vi "PathPlanner_Path_LoadPath.vi"(8 "Reversed":bool, 9 "MaxAcceleration":dbl, 10 "MaxVelocity":dbl, 11 "FileName":string="path1.path") -> (0 "error out":errorcluster, 2 "PathPlannerWayPoints":T10[](array[typedef]) {"HolonomicRotation"."SIN" format="%13.4f"; "HolonomicRotation"."COS" format="%13.4f"; "HolonomicRotation"."VALUE" format="%13.4f"; "NextControl"."Y" format="%14.3f"; "NextControl"."X" format="%14.3f"; "PrevControl"."Y" format="%14.3f"; "PrevControl"."X" format="%14.3f"; "AnchorPoint"."Y" format="%14.3f"; "AnchorPoint"."X" format="%14.3f"}, 3 "PathPlannerPath":T1={"BezierPoints"=[], "PreviewStartingRotation"={"VALUE"=0.0, "COS"=1.0, "SIN"=0.0}, "Reversed"=FALSE, "RotationTargets"=[], "ConstraintZones"=[], "EventMarkers"=[], "GlobalConstraints"={"MaxVelocityMps;"=0.0, "MaxAccelerationMpsSq;"=0.0, "MaxAngularVelRadPsEc;"=0.0, "MaxAngularAccRadPSecSq"=0.0, "Exists"=FALSE}, "GoalEndState"={"Velocity"=0.0, "Rotation"={"VALUE"=0.0, "COS"=1.0, "SIN"=0.0}}, "AllPoints"=[]} {"AllPoints"."HolonomicRotation"."SIN" format="%13.4f"; "AllPoints"."HolonomicRotation"."COS" format="%13.4f"; "AllPoints"."HolonomicRotation"."VALUE" format="%13.4f"; "AllPoints"."Position"."Y" format="%14.3f"; "AllPoints"."Position"."X" format="%14.3f"; "GoalEndState"."Rotation"."SIN" format="%13.4f"; "GoalEndState"."Rotation"."COS" format="%13.4f"; "GoalEndState"."Rotation"."VALUE" format="%13.4f"; "RotationTargets"."target"."SIN" format="%13.4f"; "RotationTargets"."target"."COS" format="%13.4f"; "RotationTargets"."target"."VALUE" format="%13.4f"; "PreviewStartingRotation"."SIN" format="%13.4f"; "PreviewStartingRotation"."COS" format="%13.4f"; "PreviewStartingRotation"."VALUE" format="%13.4f"; "BezierPoints"."Y" format="%14.3f"; "BezierPoints"."X" format="%14.3f"}, 4 "Full Filename":string)   [LabVIEW 2019, in "PathPlanner24.lvlib"]
doc: "Load a path file from storage. This loads the waypoints from a file and calculates the trajectory states. It handles combining separate paths when reversal is flagged.\n\nInputs:\n - FileName -- The name of the path to load. Absolute or relative.\n - maxVel -- Max velocity of the path\n - maxAccel -- Max velocity of the path\n - reversed -- Should the robot follow the path reversed\n\nOutputs:\n - PathPlanner Trajectory -- The generated path (path planner trajectory) can be converted to trajectory)\n - Error -- error cluster\n\nNote:\n -- Default path for roboRIO is /home/lvuser/natinst/LabVIEW Data\n -- Default path for Windows is: %USERPROFILE%\\Documents\\LabVIEW Data"
uses:
  PathPlanner24.lvlib
  <vilib>/Rock Robotics/WPI/ThirdParty/JAS_Junk/TrajLib/TypeDef/TRANSLATION2D.ctl
  <vilib>/Rock Robotics/WPI/ThirdParty/JAS_Junk/TrajLib/Trajectory_Library.lvlib
  <vilib>/Rock Robotics/WPI/ThirdParty/JAS_Junk/TrajLib/TypeDef/ROTATION2D.ctl
  TypeDef/PathPlannerWaypoint.ctl
  TypeDef/PathPlannerTrajectoryState.ctl
  TypeDef/PathPlannerTrajectory.ctl
  TypeDef/PathPlannerPathConstraints.ctl
  TypeDef/PathPlannerRotationTarget.ctl
  TypeDef/PathPlannerConstraintsZone.ctl
  TypeDef/PathPlannerEventMarker.ctl
  TypeDef/PathPlannerGoalEndState.ctl
  TypeDef/PathPlannerPathPoint.ctl
  TypeDef/PathPlannerPath.ctl
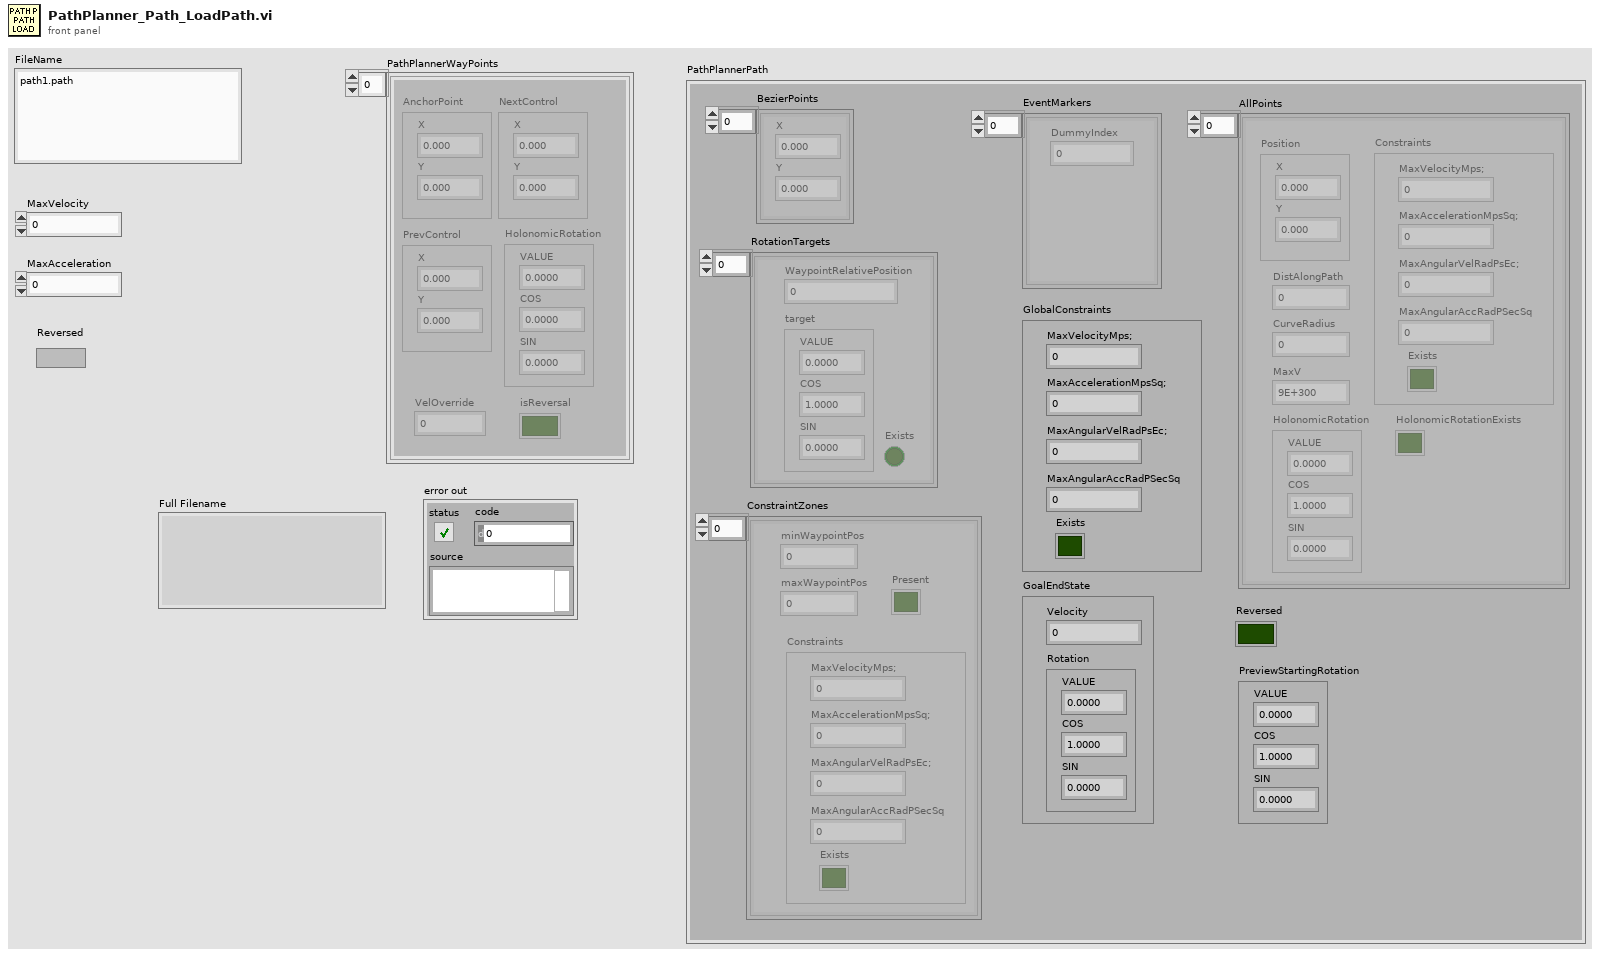
[diagram p1: front panel]
types:
  T1 = typedef "PathPlanner24.lvlib/PathPlannerPath.ctl" = cluster{"BezierPoints":T2[], "PreviewStartingRotation":T3, "Reversed":bool, "RotationTargets":T4[], "ConstraintZones":T5[], "EventMarkers":T7[], "GlobalConstraints":T6, "GoalEndState":T8, "AllPoints":T9[]}
  T2 = typedef "Trajectory_Library.lvlib/TRANSLATION2D.ctl" = cluster{"X":dbl, "Y":dbl}
  T3 = typedef "Trajectory_Library.lvlib/ROTATION2D.ctl" = cluster{"VALUE":dbl, "COS":dbl, "SIN":dbl}
  T4 = typedef "PathPlanner24.lvlib/PathPlannerRotationTarget.ctl" = cluster{"target":T3, "WaypointRelativePosition":dbl, "Exists":bool}
  T5 = typedef "PathPlanner24.lvlib/PathPlannerConstraintsZone.ctl" = cluster{"minWaypointPos":dbl, "maxWaypointPos":dbl, "Constraints":T6, "Present":bool}
  T6 = typedef "PathPlanner24.lvlib/PathPlannerPathConstraints.ctl" = cluster{"MaxVelocityMps;":dbl, "MaxAccelerationMpsSq;":dbl, "MaxAngularVelRadPsEc;":dbl, "MaxAngularAccRadPSecSq":dbl, "Exists":bool}
  T7 = typedef "PathPlanner24.lvlib/PathPlannerEventMarker.ctl" = cluster{"DummyIndex":i32}
  T8 = typedef "PathPlanner24.lvlib/PathPlannerGoalEndState.ctl" = cluster{"Velocity":dbl, "Rotation":T3}
  T9 = typedef "PathPlanner24.lvlib/PathPlannerPathPoint.ctl" = cluster{"Position":T2, "HolonomicRotation":T3, "DistAlongPath":dbl, "CurveRadius":dbl, "MaxV":dbl, "Constraints":T6, "HolonomicRotationExists":bool}
  T10 = typedef "PathPlanner24.lvlib/PathPlannerWaypoint.ctl" = cluster{"AnchorPoint":T2, "PrevControl":T2, "NextControl":T2, "HolonomicRotation":T3, "VelOverride":dbl, "isReversal":bool}
  T11 = typedef "PathPlanner24.lvlib/PathPlannerTrajectory.ctl" = cluster{"States":T12[]}
  T12 = typedef "PathPlanner24.lvlib/PathPlannerTrajectoryState.ctl" = cluster{"TimeSeconds":dbl, "VelocityMPS":dbl, "AccerationMpsSq":dbl, "HeadingAngularVelRadPerSec":dbl, "PositionMeters":T2, "Heading":T3, "TargetHolonomicRotation":T3, "CurvatureRadPerMeter":dbl, "DeltaPos":dbl, "PathPlannerConstraints":T6}
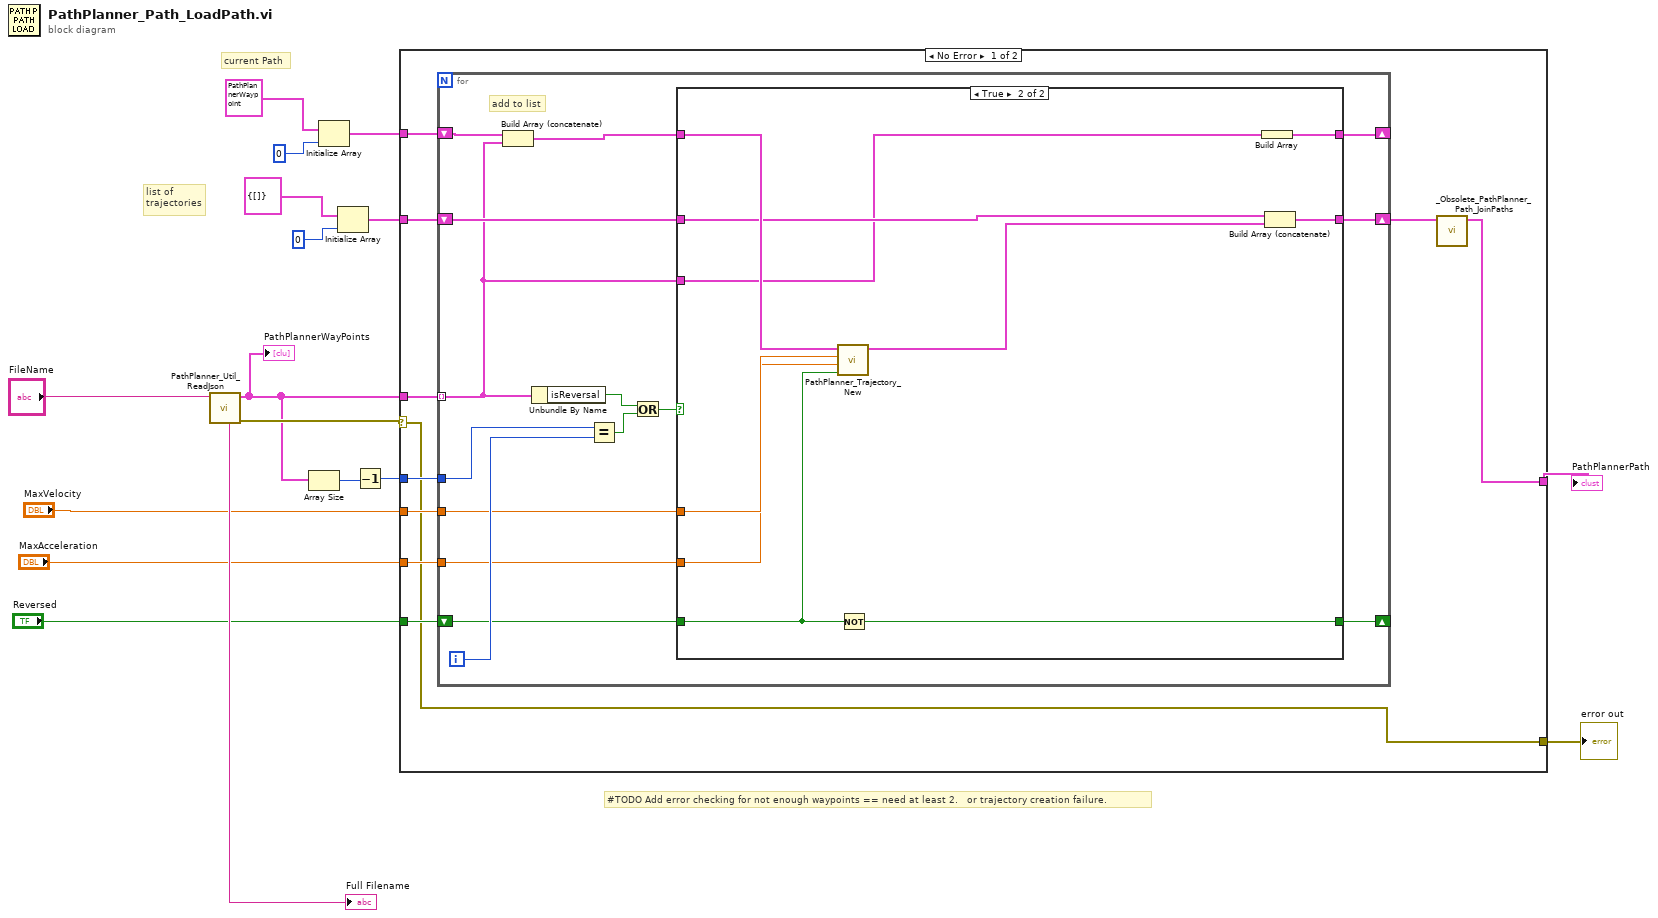
[diagram p0: block diagram]
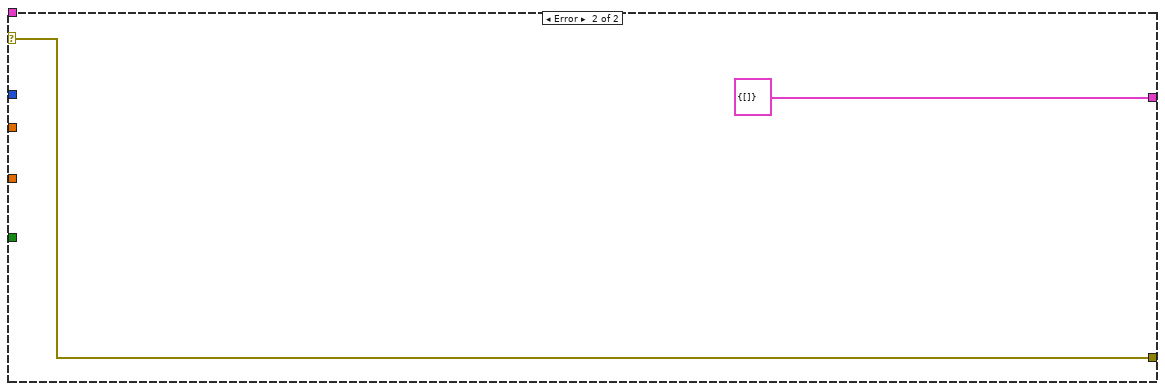
[diagram p3: hidden frame]
diagram:
  # "#TODO Add error checking for not enough waypoints == need at least 2.   or trajectory creation failure."
  # "list of \ntrajectories"
  # "current Path"
  n1 = call "PathPlanner_Util_ReadJson.vi"("FileName"="FileName") -> ("error out"=w15:errorcluster, "PathPlannerWayPoints"=w3:T10[], "Full Filename"=→"Full Filename":string)  [unwired: 8 in]
  "PathPlannerWayPoints" <- w3
  n2 = Array Size(array=w3) -> (size(s)=w9:i32)
  n3 = Initialize Array(T10 {"AnchorPoint"={"X"=0.0, "Y"=0.0}, "PrevControl"={"X"=0.0, "Y"=0.0}, "NextControl"={"X"=0.0, "Y"=0.0}, "HolonomicRotation"={"VALUE"=0.0, "COS"=1.0, "SIN"=0.0}, "VelOverride"=0.0, "isReversal"=FALSE} ("PathPlannerWaypoint"), 0 ("dimension size")) -> (w12:T10[])
  n4 = Initialize Array(T11 {"States"=[]} ("PathPlannerTrajectory"), 0 ("dimension size")) -> (w7:T11[])
  n5 = Decrement(x=w9) -> (x-1=w8:i32)
  n6 = case shown="No Error" w15 {
    selector: w15 -> [w20 w56]
    tunnel: w12 -> [w27 _]
    tunnel: w3 -> [w26 _]
    tunnel: w8 -> [w25 _]
    tunnel: w7 -> [w24 _]
    tunnel: "MaxVelocity" -> [w23 _]
    tunnel: "MaxAcceleration" -> [w22 _]
    tunnel: "Reversed" -> [w21 _]
    tunnel: [w18 T11 {"States"=[]} ("PathPlannerTrajectory")] -> w2
    tunnel: [w20 w56] -> w1
    frame No Error {
      n7 = for {
        shift-right: [w33] -> _
        shift-left: w27 -> [w42]
        tunnel: w26 -> [w28] mode=indexing
        tunnel: w25 -> [w39]
        shift-right: [w35] -> w19
        shift-left: w24 -> [w36]
        tunnel: w23 -> [w32]
        tunnel: w22 -> [w31]
        shift-right: [w29] -> _
        shift-left: w21 -> [w30]
        i -> [w38]
        # "add to list"
        n8 = Build Array (concatenate)(w42, w28) -> (w34:T10[])
        n9 = Unbundle By Name(w28) -> ("isReversal"=w41:bool)
        n10 = Equal?(x=w39, y=w38) -> (x = y?=w40:bool)
        n11 = Or(x=w41, y=w40) -> (x .or. y?=w37:bool)
        n12 = case shown="True" w37 {
          tunnel: w36 -> [w45 w51]
          tunnel: [w45 w52] -> w35
          tunnel: w34 -> [w44 w55]
          tunnel: [w44 w47] -> w33
          tunnel: w32 -> [_ w54]
          tunnel: w31 -> [_ w53]
          tunnel: w30 -> [w43 w48]
          tunnel: [w43 w49] -> w29
          tunnel: w28 -> [_ w46]
          frame False {
          }
          frame True {
            n13 = call "PathPlanner_Trajectory_New.vi"(8:w48, 9:w53, "StartingSpeeds"=w54, "Path"=w55) -> ("PathPlannerTrajectory"=w50:T11)  [unwired: 7 in]
            n14 = Not(x=w48) -> (.not. x?=w49:bool)
            n15 = Build Array(w46) -> (w47:T10[])
            n16 = Build Array (concatenate)(w51, w50) -> (w52:T11[])
          }
        }
      }
      n17 = call "_Obsolete_PathPlanner_Path_JoinPaths.vi"("in Trajectories"=w19) -> ("out PathPlannerTrajectory"=w18:T11)  [unwired: 10 in]
    }
    frame Error {
    }
  }
  "error out" <- w1
  "PathPlannerPath" <- w2
